vi "bit compare 1_0_dontcare_SAVE.vi"(9 "Input":bool[](array[boolean]), 10 "Match This Pattern":enum16{"TRUE", "FALSE", "DONTCARE"}[](array[ring])=[enum."TRUE", enum."DONTCARE", enum."TRUE", enum."DONTCARE", enum."FALSE", enum."TRUE", enum."FALSE"]) -> (2 "x = y?":bool)   [LabVIEW 2018]
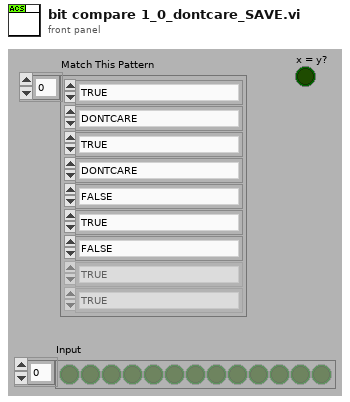
[diagram p1: front panel]
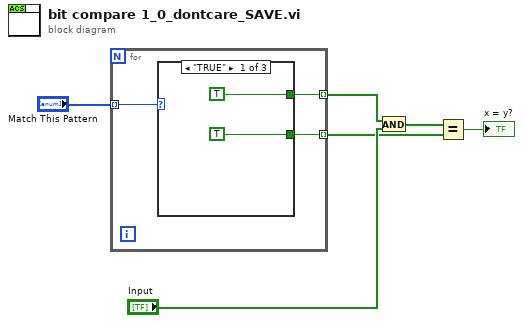
[diagram p0: block diagram]
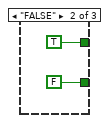
[diagram p2: hidden frame]
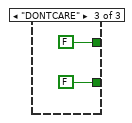
[diagram p3: hidden frame]
diagram:
  n1 = for {
    tunnel: "Match This Pattern" -> [w9] mode=indexing
    tunnel: [w8] -> w5 mode=indexing
    tunnel: [w7] -> w2 mode=indexing
    n2 = case shown="\"TRUE\"" w9 {
      tunnel: [TRUE TRUE FALSE] -> w8
      tunnel: [TRUE FALSE FALSE] -> w7
      frame "TRUE" {
      }
      frame "FALSE" {
      }
      frame "DONTCARE" {
      }
    }
  }
  n3 = And(x=w5, y="Input") -> (x .and. y?=w3:bool[])
  n4 = Equal?(x=w3, y=w2) -> (x = y?=→"x = y?":bool)
